vi "NI9263_simpleUI.vi"() -> ()   [LabVIEW 2020]
uses:
  TYPEDEF/NI9263_TD_Method.ctl
panel:
  in  "Channels NI9263":tag="cDAQ1Mod4/ao1"
  in  "Stop":bool
  in  "V in Ch":dbl=1.6
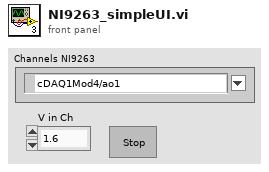
[diagram p1: front panel]
types:
  T1 = typedef "NI9263_TD_Method.ctl" = enum16{"NO_OP", "INIT", "SET", "GET", "CLOSE"}
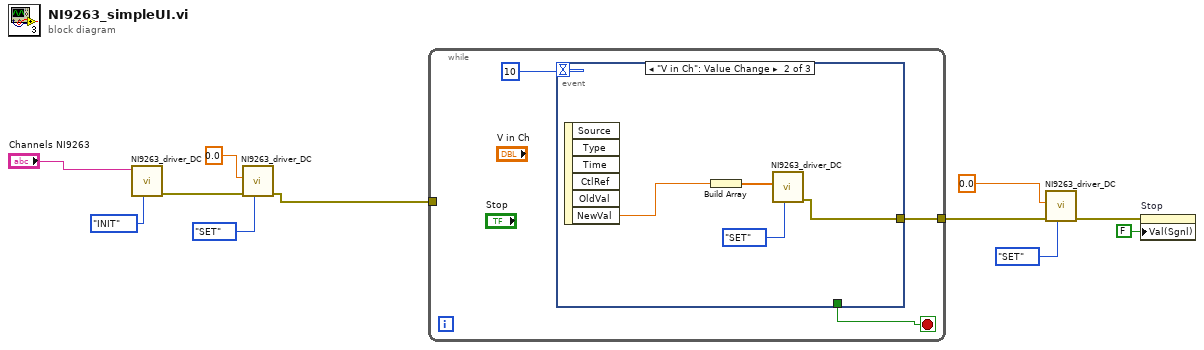
[diagram p0: block diagram]
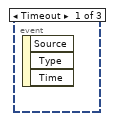
[diagram p2: hidden frame]
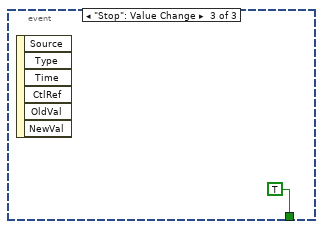
[diagram p3: hidden frame]
diagram:
  n1 = call "NI9263_driver_DC.vi"("METHOD"=NI9263_TD_Method."INIT", "Channels NI9263"="Channels NI9263") -> ("error out"=w8:errorcluster)  [unwired: 9 in]
  n2 = call "NI9263_driver_DC.vi"("METHOD"=NI9263_TD_Method."SET", "error in (no error)"=w8, "Channel Values"=0.0) -> ("error out"=w2:errorcluster)  [unwired: 8 in]
  n3 = while {
    tunnel: [w12] -> w6
    tunnel: w2 -> [_]
    stop <- w13 stop-if-true
    n4 = event shown="[1] \"V in Ch\": Value Change" {
      selector: _ -> [_ _ _]
      dyn-events: _ -> [_ _ _]
      timeout: 10 -> [_ _ _]
      tunnel: [_ _ TRUE] -> w13
      tunnel: [_ w17 _] -> w12
      event Timeout {
        n5 = event-data() -> ()  [unwired: 1 in, 3 out]
      }
      event "V in Ch": Value Change {
        n6 = event-data() -> ("NewVal"=w15:dbl)  [unwired: 1 in, 5 out]
        n7 = Build Array(w15) -> (w16:dbl[])
        n8 = call "NI9263_driver_DC.vi"("METHOD"=NI9263_TD_Method."SET", "Channel Values"=w16) -> ("error out"=w17:errorcluster)  [unwired: 9 in]
      }
      event "Stop": Value Change {
        n9 = event-data() -> ()  [unwired: 1 in, 6 out]
      }
    }
  }
  n10 = call "NI9263_driver_DC.vi"("METHOD"=NI9263_TD_Method."SET", "error in (no error)"=w6, "Channel Values"=0.0) -> ("error out"=w5:errorcluster)  [unwired: 8 in]
  n11 = property on="Stop" class="Bool (strict)"(error in=w5, "Val(Sgnl)"=FALSE ("Value (Signaling)")) -> ()  [unwired: 1 in, 2 out]
